vi "Device Settings.vi"(8 "error in":errorcluster, 11 "Class Objects In":T1) -> (0 "error out":errorcluster, 3 "Class Objects Out":T1)   [LabVIEW 2011]
uses:
  Controls/Class Objects.ctl
  Modules/File/Configuration/Configuration.lvclass
  Modules/Hardware/Mass Flow Controller/Mass Flow Controller.lvclass
  Modules/Hardware/Valve Controller/Valve Controller.lvclass
  Modules/Hardware/Power Supply/Power Supply.lvclass
  Modules/Hardware/Vapour Generator/Vapour Generator.lvclass
  Modules/Hardware/PID/PID.lvclass
  Modules/Hardware/Multimeter/Multimeter.lvclass
  Modules/File/TDMS/TDMS.lvclass
  Modules/Hardware/Power Supply/Source Mode.ctl
  Modules/Hardware/Power Supply/Source Units.ctl
  Modules/Hardware/Power Supply/Protection Limits.ctl
  Modules/Hardware/Power Supply/Voltage Units.ctl
  Modules/Hardware/Power Supply/Current Units.ctl
  Modules/Hardware/Aalborg GFC17/Flow Rate.ctl
  Modules/Hardware/Mass Flow Controller/Valve Status.ctl
  Modules/Hardware/Valve Controller/Valve Assembly.ctl
  Modules/Hardware/Valve Controller/Status.ctl
  Modules/Hardware/Agilent 3458A/Measurement Configuration.ctl
  Modules/Hardware/Agilent 3458A/Measurement Integration.ctl
  Modules/Hardware/Baseline Mocon piD-Tech plus/Settings.ctl
  Modules/Hardware/INL PID/Settings.ctl
  Modules/Hardware/Owlstone GEN-SYS/Permeation Tube.ctl
  Modules/Hardware/Owlstone GEN-SYS/Permeation Tube Gas.ctl
  Modules/Hardware/Owlstone GEN-SYS/Gen-Sys Setpoints.ctl
  Modules/Hardware/Vapour Generator/Gas Output.ctl
  Functional Global Data/Device Params Global.ctl
  Controls/Detector Type.ctl
  Controls/User Interface Action.ctl
  Controls/Devices.ctl
  Functional Global Data/Status Bar.ctl
  Modules/Hardware/Owlstone GEN-SYS/Owlstone GEN-SYS.lvclass
  Modules/Hardware/Agilent 3458A/Agilent 3458A.lvclass
  Modules/Hardware/Mass Flow Controller/Flow Rate Units.ctl
  Modules/Hardware/Valve Controller/Valves.ctl
  Modules/Hardware/Aalborg GFC17/Aalborg GFC17.lvclass
  Modules/Hardware/Baseline Mocon piD-Tech plus/Baseline Mocon piD-Tech plus.lvclass
  Modules/Hardware/INL PID/INL PID.lvclass
panel:
  in  "?":T2(tab)
  out "Gas Output":T3={"Concentration (ppm)"=inf, "Flow Rate (ml/min)"=0.0, "Relative Humidity (%)"=-1.0} {"Relative Humidity (%)" format="%#.4g"; "Flow Rate (ml/min)" format="%#.0f"; "Concentration (ppm)" format="%#.2g"}
  in  "Owlstone GEN-SYS Setpoints":T4={"OVG-4"={"Oven Temperature"=50, "Sample Flow Rate"=250, "Split Flow Status"=0, "Split Flow Rate"=0}, "OHG-4"={"Wet Air Flow"=500}} {"OHG-4"."Wet Air Flow" min=300 max=3000 scale=300.0..3000.0; "OVG-4"."Split Flow Status" items=["Closed", "Open"]; "OVG-4"."Split Flow Rate" min=300 max=3000 scale=50.0..3000.0; "OVG-4"."Sample Flow Rate" min=50 max=500 scale=50.0..500.0; "OVG-4"."Oven Temperature" min=25 max=100 scale=25.0..100.0}
  in  "Owlstone Permeation Tube":T5={"Tube"=enum."Ammonia 29 Sep 2012", "Molecular Weight"=56.106, "Calibration Temperature\n(Celcius)"=50, "Permeation Rate \n(ng/min)"=1539} {"Molecular Weight" min=0.0 format="%#.3g"; "Permeation Rate \n(ng/min)" min=0; "Calibration Temperature\n(Celcius)" min=0}
  in  "INL PID Settings":T7 caption="INL PID"
  in  "B-M PID Settings":T8 caption="Baseline Mocon piD-TECH plus"
  in  "Power Supply Output":bool caption="Output"
  in  "Power Supply Apply":bool
  in  "Power Supply Limits":T9 caption="Limits"
  in  "Power Supply Source Value Units":T12 caption="Source Value Units"
  in  "Power Supply Source Value":dbl caption="Source Value"
  in  "Power Supply Source Mode":T13 caption="Source Mode"
  in  "Agilent 3458A Measurement Integration":T14={"Power Line Cycles"=10.0} caption="Measurement Integration"
  in  "Agilent 3458A Multimeter Measurement Configuration":T15 caption="Measurement Configuration"
  in  "MFC Valve Status":T16=enum."Closed" caption="Valve Status"
  in  "MFC Flow Rate":T17 caption="Flow Rate" min=0.0 max=200.0 scale=0.0..200.0
  in  "Valves Open All":bool
  in  "Valves Close All":bool
  in  "Valve Assembly":T18 {"Valve 5" items=["Closed", "Open"]; "Valve 4" items=["Closed", "Open"]; "Valve 3" items=["Closed", "Open"]; "Valve 2" items=["Closed", "Open"]; "Valve 1" items=["Closed", "Open"]}
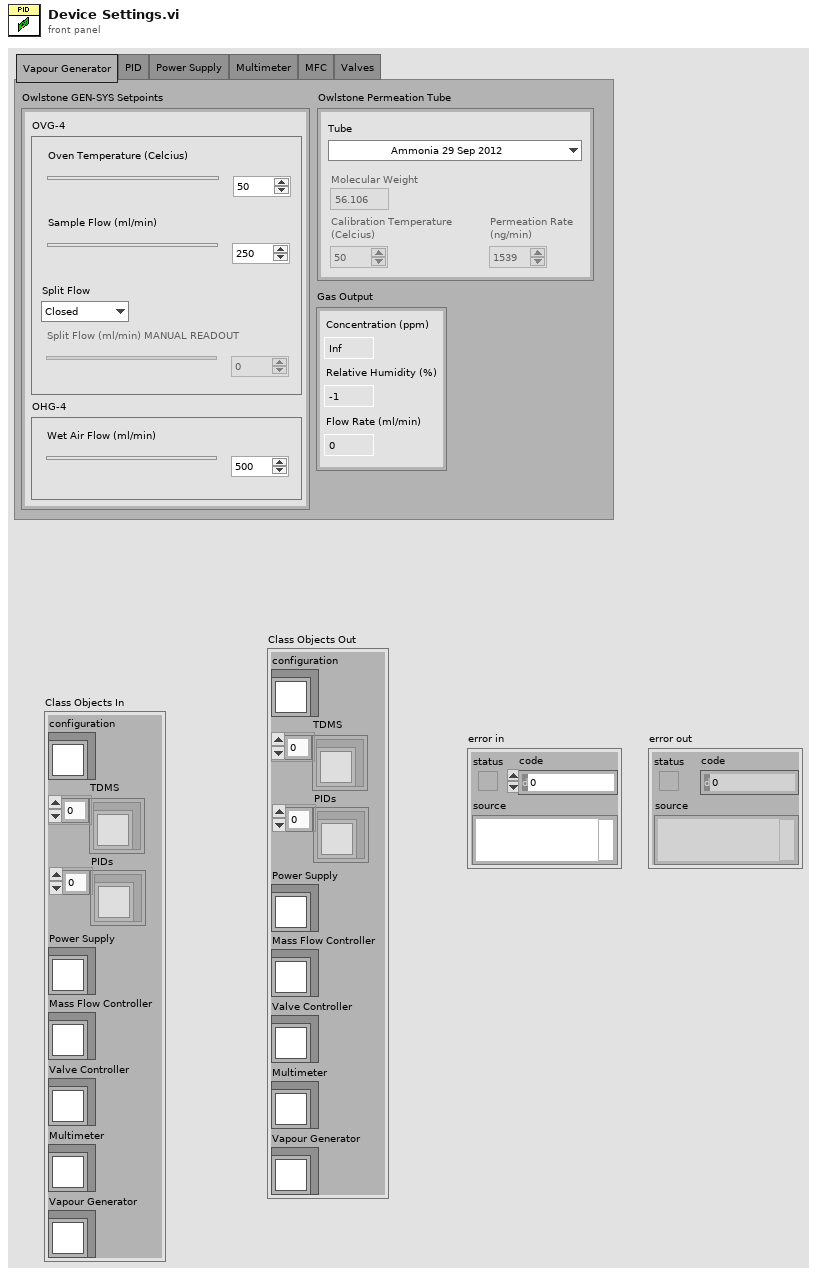
[diagram p1: front panel]
types:
  T1 = typedef "Class Objects.ctl" = cluster{"configuration":refnum<class "Configuration.lvclass">, "TDMS":refnum<class "TDMS.lvclass">[], "Power Supply":refnum<class "Power Supply.lvclass">, "Mass Flow Controller":refnum<class "Mass Flow Controller.lvclass">, "Valve Controller":refnum<class "Valve Controller.lvclass">, "Multimeter":refnum<class "Multimeter.lvclass">, "Vapour Generator":refnum<class "Vapour Generator.lvclass">, "PIDs":refnum<class "PID.lvclass">[]}
  T2 = enum32{"Vapour Generator", "PID", "Power Supply", "Multimeter", "MFC", "Valves"}
  T3 = typedef "Vapour Generator.lvclass/Gas Output.ctl" = cluster{"Concentration (ppm)":dbl, "Flow Rate (ml/min)":dbl, "Relative Humidity (%)":dbl}
  T4 = typedef "Owlstone GEN-SYS.lvclass/Gen-Sys Setpoints.ctl" = cluster{"OVG-4":cluster{"Oven Temperature":i32, "Sample Flow Rate":i32, "Split Flow Status":u16, "Split Flow Rate":i32}, "OHG-4":cluster{"Wet Air Flow":i32}}
  T5 = typedef "Owlstone GEN-SYS.lvclass/Permeation Tube.ctl" = cluster{"Tube":T6, "Molecular Weight":dbl, "Calibration Temperature\n(Celcius)":i32, "Permeation Rate \n(ng/min)":i32}
  T6 = typedef "Owlstone GEN-SYS.lvclass/Permeation Tube Gas.ctl" = enum16{"Isobutylene 27 Nov 2012", "Ammonia 29 Sep 2012", "DMMP Tube A 3 July 2014", "DMMP Tube B 3 July 2014"}
  T7 = typedef "INL PID.lvclass/Settings.ctl" = cluster{"Sampling Frequency":dbl, "Integration Time":dbl, "Integration Periods":u8, "Grid Voltage":dbl}
  T8 = typedef "Baseline Mocon piD-Tech plus.lvclass/Settings.ctl" = cluster{"Detector Sampling Frequency":dbl}
  T9 = typedef "Power Supply.lvclass/Protection Limits.ctl" = cluster{"Voltage Limit":dbl, "Voltage Limit Units":T10, "Current Limit":dbl, "Current Limit Units":T11, "Voltage Trip/Cmpl":dbl, "Voltage Trip/Cmpl Units":T10, "Current Trip/Cmpl":dbl, "Current Trip/Cmpl Units":T11}
  T10 = typedef "Power Supply.lvclass/Voltage Units.ctl" = enum16{"volts", "millivolts", "microvolts"}
  T11 = typedef "Power Supply.lvclass/Current Units.ctl" = enum16{"amps", "milliamps", "microamps", "nanoamps"}
  T12 = typedef "Power Supply.lvclass/Source Units.ctl" = enum16{"volts", "millivolts", "microvolts", "amps", "milliamps", "microamps", "nanoamps"}
  T13 = typedef "Power Supply.lvclass/Source Mode.ctl" = enum16{"Volts", "Current"}
  T14 = typedef "Agilent 3458A.lvclass/Measurement Integration.ctl" = cluster{"Power Line Cycles":dbl}
  T15 = typedef "Agilent 3458A.lvclass/Measurement Configuration.ctl" = cluster{"Function":enum16{"DC Voltage", "AC Voltage", "AC + DC Voltage", "DC Current", "AC Current", "AC + DC Current", "2-Wire Resistance", "4-Wire Resistance", "Frequency", "Period", "Direct Sampling DC", "Direct Sampling AC", "Sub-Sampling DC", "Sub-Sampling AC"}, " Manual Resolution":enum16{"4.5", "5.5", "6.5", "7.5", "8.5"}, "Frequency Source":enum16{"AC + DC Current", "AC + DC Voltage", "AC Current", "AC Voltage"}, "Auto Range":enum16{"OFF", "ON", "ONCE"}}
  T16 = typedef "Mass Flow Controller.lvclass/Valve Status.ctl" = enum16{"Open", "Closed"}
  T17 = typedef "Aalborg GFC17.lvclass/Flow Rate.ctl" = dbl
  T18 = typedef "Valve Controller.lvclass/Valve Assembly.ctl" = cluster{"Valve 1":T19, "Valve 2":T19, "Valve 3":T19, "Valve 4":T19, "Valve 5":T19}
  T19 = typedef "Valve Controller.lvclass/Status.ctl" = u16
  T20 = typedef "Device Params Global.ctl" = enum16{"Initialize", "Get Device Settings", "Get Device Connections", "Set Device Settings", "Set Device Connections", "Get All Device Properties"}
  T21 = typedef "Device Connections.ctl" = cluster{"Detector":cluster{"Detector Type":T22, "Connection":bool, "B-M PID":T23, "INL PID Connections":T24}, "Power Supply":cluster{"Type":enum16{"Stanford Research PS350", "Keithley 2400"}, "Connection":bool, "VISA resource name":refnum<visa-resource-name>}, "Mass Flow Controller":cluster{"Type":enum16{"Aalborg GFC17"}, "Connection":bool, "Aalborg GFC17":T26}, "Valve Controller":cluster{"Type":T27, "Connection":bool, "SMC - INL":cluster{"VISA resource name":refnum<visa-resource-name>}}, "Multimeter":cluster{"Multimeter Type":T28, "Connection":bool, "VISA resource name":refnum<visa-resource-name>}, "Vapour Generator":cluster{"Type":T29, "Connection":bool, "Owlstone Gen-SYS":T30}}
  T22 = typedef "Detector Type.ctl" = enum16{"INL PID", "Baseline-Mocon piD-TECH plus"}
  T23 = typedef "Baseline Mocon piD-Tech plus.lvclass/Connections.ctl" = cluster{"AI DAQmx channel":tag}
  T24 = typedef "INL PID Connections.ctl" = cluster{"PIDs":u8, "Integrator DAQ Channels 1":T25, "Integrator DAQ Channels 2":T25}
  T25 = typedef "INL PID.lvclass/Integrator DAQmx Channels.ctl" = cluster{"V0":tag, "S1":tag, "S2":tag}
  T26 = typedef "Aalborg GFC17.lvclass/Aalborg GFC17 Connections.ctl" = cluster{"flow rate setpoint channel":tag, "flow rate reading channel":tag, "valve channel":tag}
  T27 = typedef "Valve Type.ctl" = enum16{"SMC - INL"}
  T28 = typedef "Multimeter Type.ctl" = enum16{"Agilent 3458A"}
  T29 = typedef "Vapour Generator Type.ctl" = enum16{"Owlstone GEN-SYS"}
  T30 = typedef "Owlstone GEN-SYS.lvclass/GEN-SYS Connections.ctl" = cluster{"GEN-SYS VISA resource name":refnum<visa-resource-name>, "OVG-4":cluster{"Flow Address":u8, "Temp Address":u8}, "OHG-4":cluster{"Flow Address":u8, "Easydew VISA resource name":refnum<visa-resource-name>}}
  T31 = typedef "Device Settings.ctl" = cluster{"PID":cluster{"B-M PID":T8, "INL PID":T7}, "Power Supply":cluster{"Source Value":dbl, "Source Value Units":T12, "Source Mode":T13, "Limits":T9, "Output":bool}, "Mass Flow Controller":cluster{"MFC Flow Rate":dbl, "MFC Valve Status":T16}, "Valve Controller":cluster{"Valve Assembly":T18}, "Multimeter":cluster{"Agilent 3458A":cluster{"Measurement Configuration":T15, "Measurement Integration":T14}}, "Vapour Generator":cluster{"Owlstone Permeation Tube":T5, "Owlstone GEN-SYS Setpoints":T4}}
  T32 = enum8{"Enabled", "Disabled", "Disabled and Grayed Out"}
  T33 = cluster{"Valve 1":T19, "Valve 2":T19, "Valve 3":T19, "Valve 4":T19, "Valve 5":T19}
  T34 = typedef "User Interface Action.ctl" = enum16{"Initialize", "Data Acquisition Disable", "Data View Disable", "Sample Set", "Sample Set 2D Data", "Sample Set x0 & dx", "Sample Add", "Sample Set Cursor", "Sample Set Offset & Multiplier", "Sample Set Axis Labels", "Sample Parameters Disabled", "Sample Parameters Update", "Run Update", "Run Set Offset & Multiplier", "Run Set Axis Labels", "Run Set Cursor", "Run Set Disabled", "Run Parameters Update", "Run Parameters Disabled", "Run Number Set", "Run Number Set Range", "Run Number Set Disabled", "Sample Number Set", "Sample Number Set Range", "Notes Set Value", "Update Plot", "Set Plot Parameters", "Update Concentration Plot", "Time Set", "Clear DAQ Display", "Clear Analysis Display", "Status Bar Set", "Progress Bar Set", "Display Mode Set", "Experiment Type Set", "Analysis Plot Average Set", "Stop"}
  T35 = typedef "Devices.ctl" = enum16{"Detector", "Mass Flow Controller", "Power Supply"}
  T36 = typedef "Status Bar.ctl" = enum16{"Insert Into Status Bar", "Get Status Bar", "Initialize"}
  T37 = typedef "Mass Flow Controller.lvclass/Flow Rate Units.ctl" = enum16{"ml/min"}
  T38 = enum16{"Stanford Research PS350", "Keithley 2400"}
  T39 = cluster{"Tube":T6, "Molecular Weight":dbl, "Calibration Temperature\n(Celcius)":i32, "Permeation Rate \n(ng/min)":i32}
  T40 = typedef "Valve Controller.lvclass/Valves.ctl" = u16
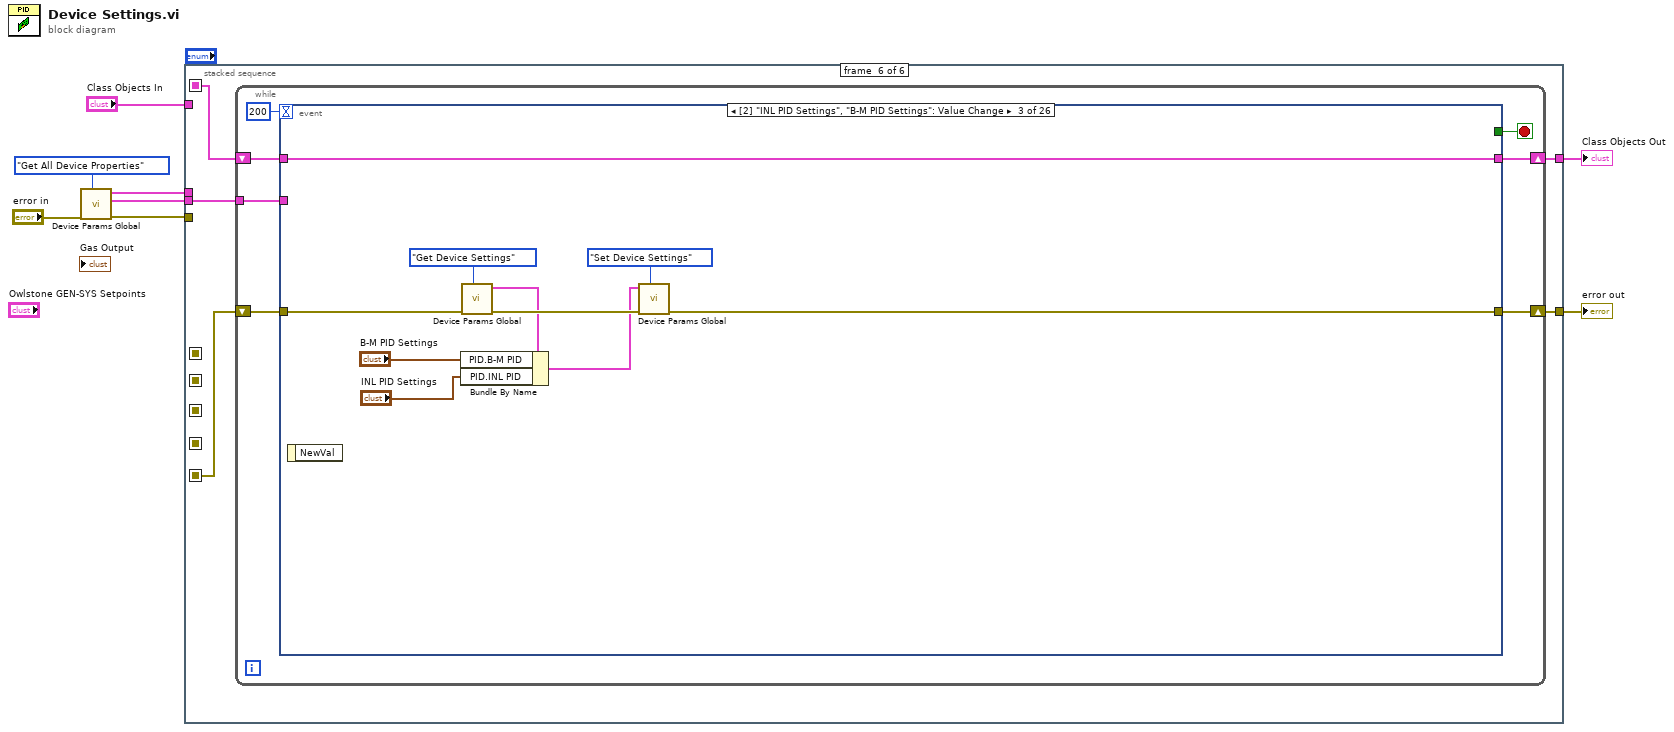
[diagram p0: block diagram]
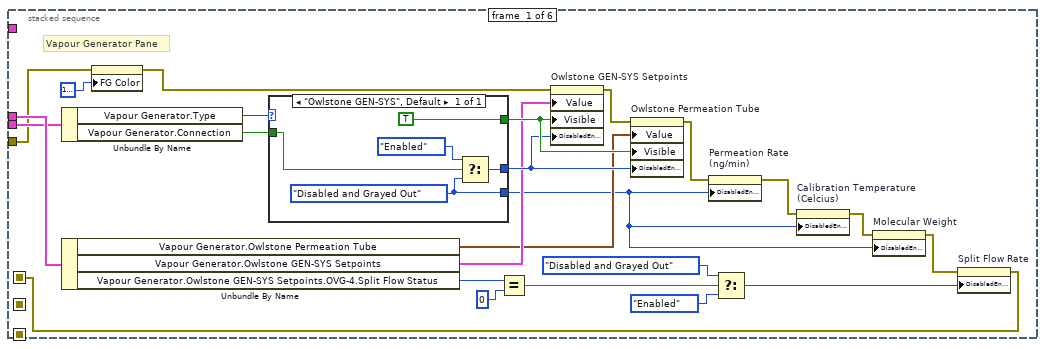
[diagram p2: hidden frame]
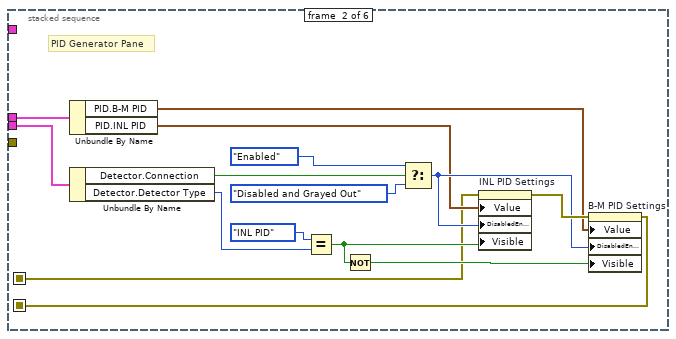
[diagram p3: hidden frame]
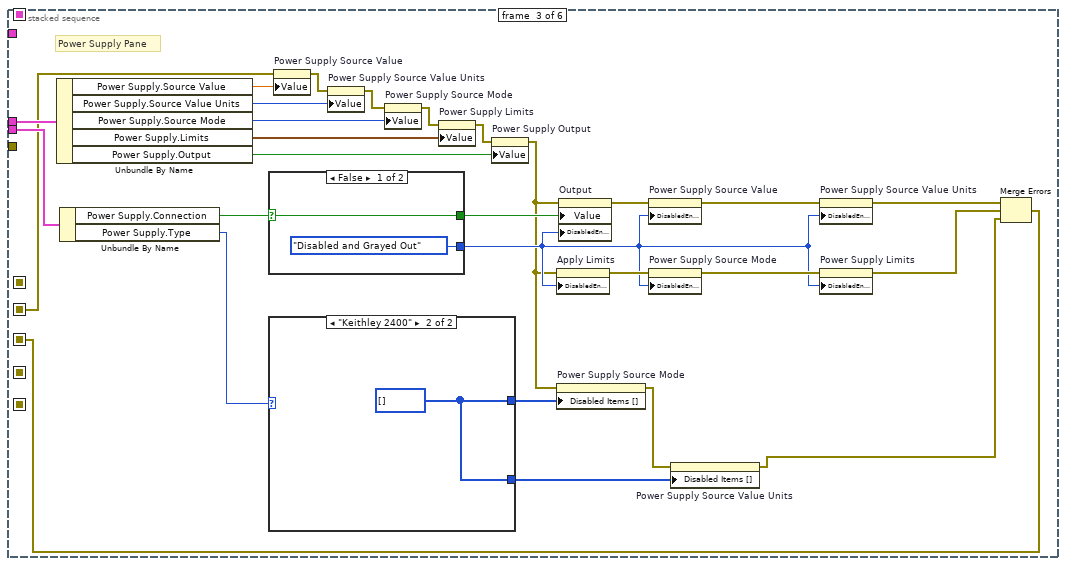
[diagram p4: hidden frame]
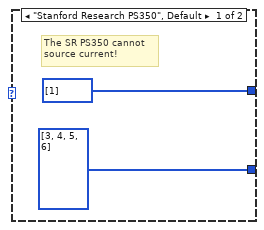
[diagram p5: hidden frame]
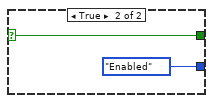
[diagram p6: hidden frame]
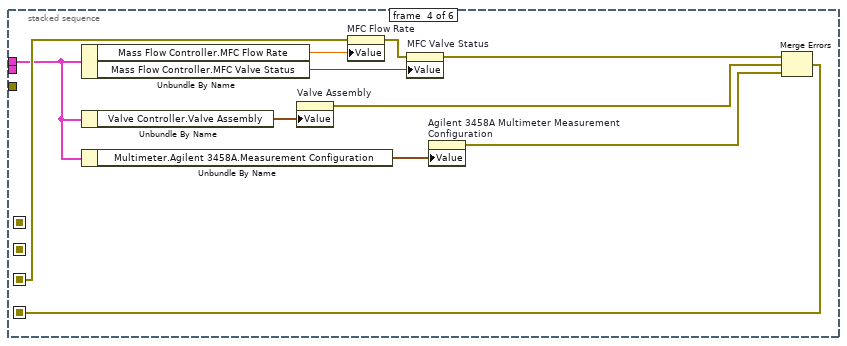
[diagram p7: hidden frame]
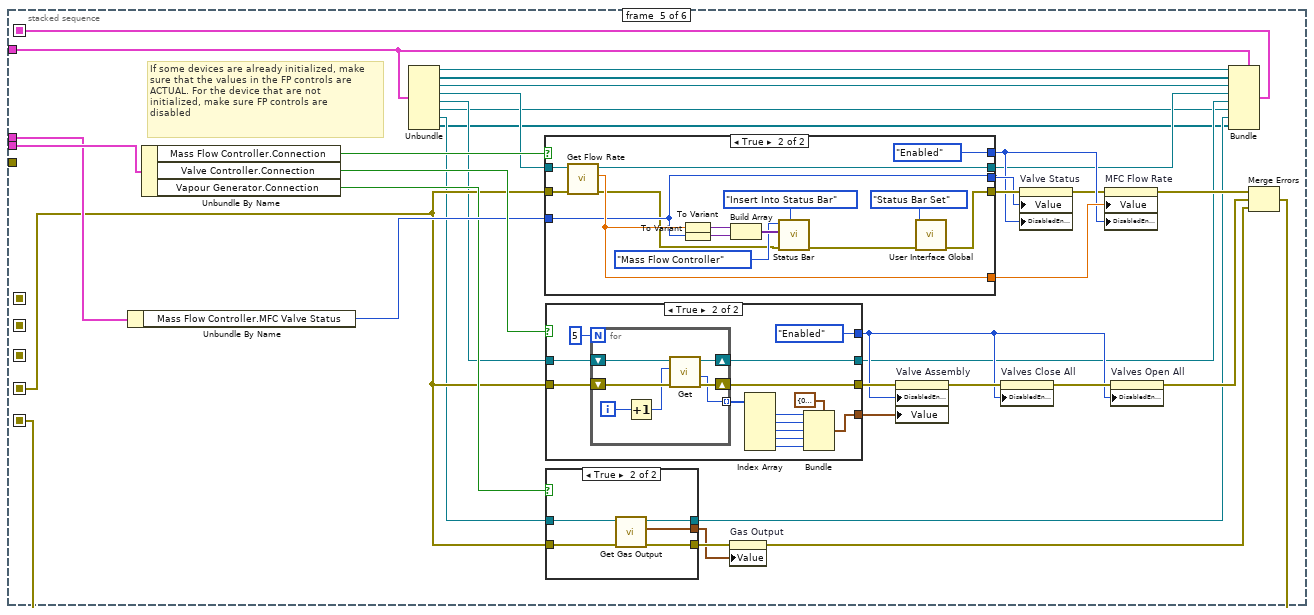
[diagram p8: hidden frame]
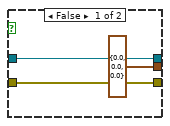
[diagram p9: hidden frame]
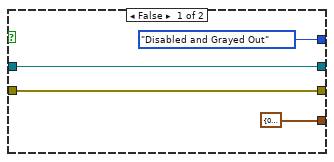
[diagram p10: hidden frame]
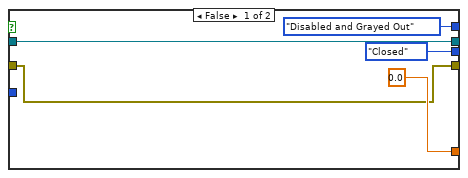
[diagram p11: hidden frame]
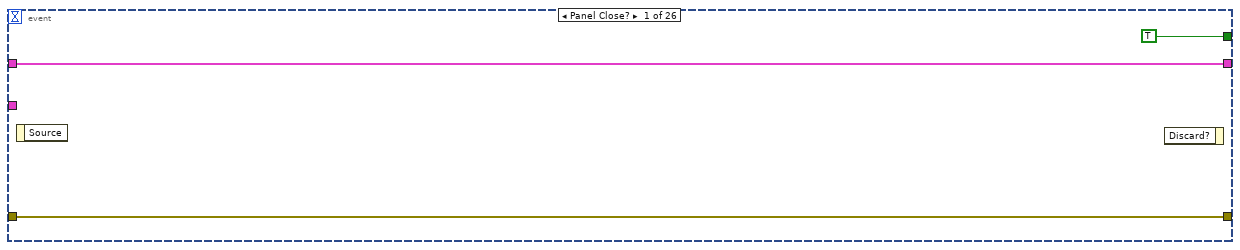
[diagram p12: hidden frame]
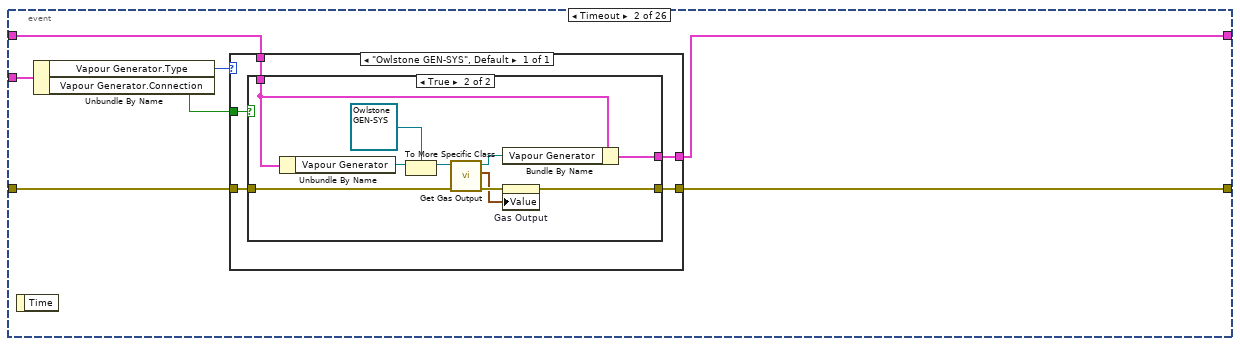
[diagram p13: hidden frame]
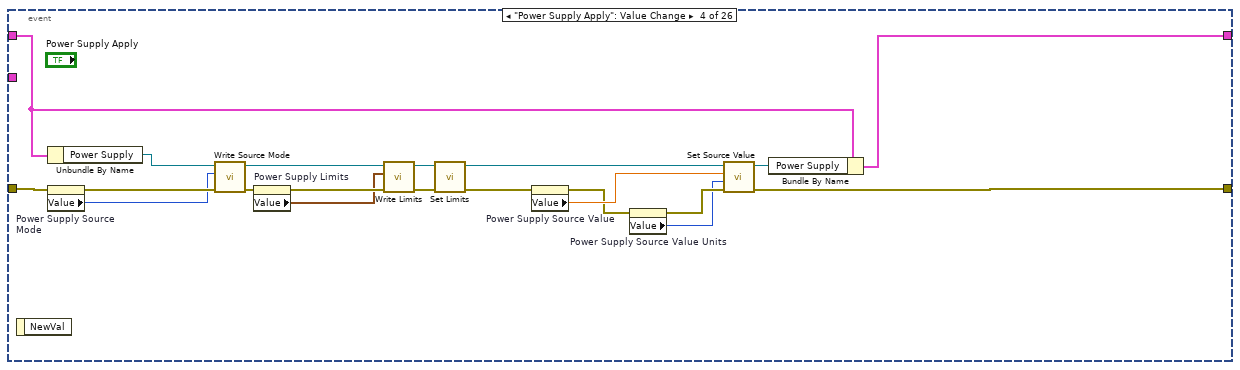
[diagram p15: hidden frame]
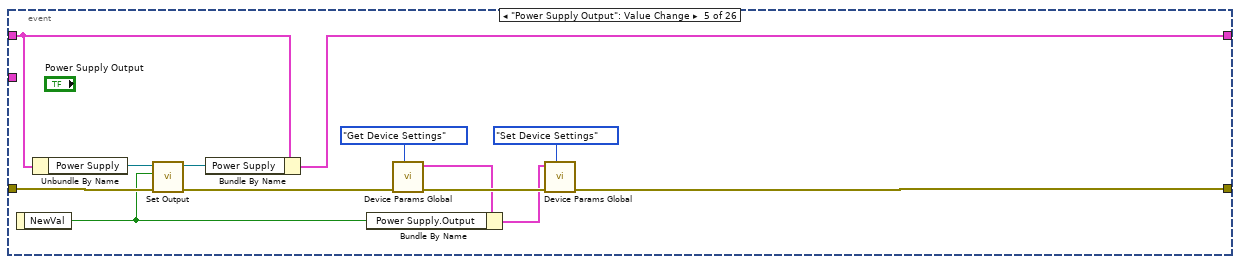
[diagram p16: hidden frame]
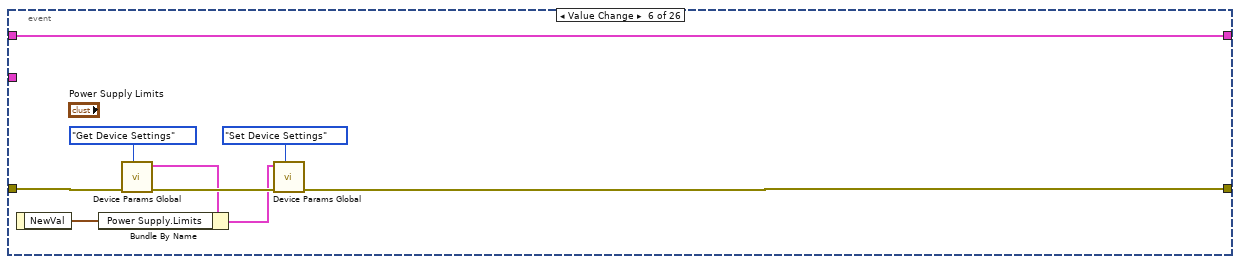
[diagram p17: hidden frame]
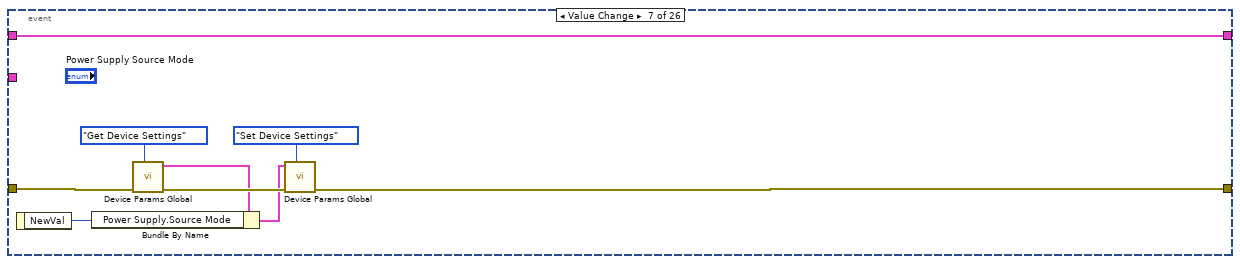
[diagram p18: hidden frame]
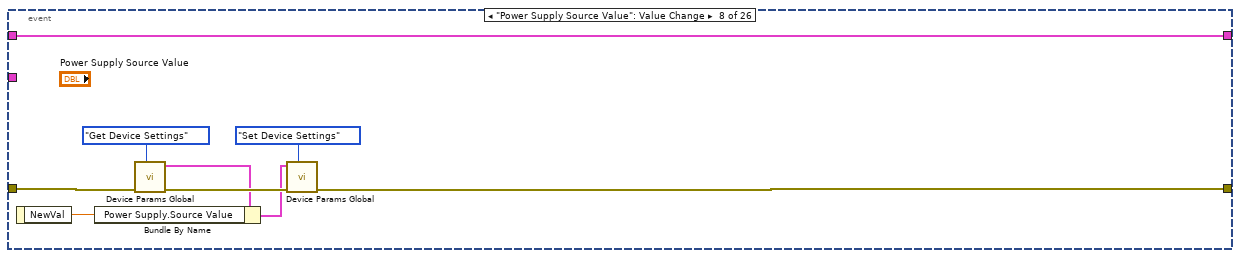
[diagram p19: hidden frame]
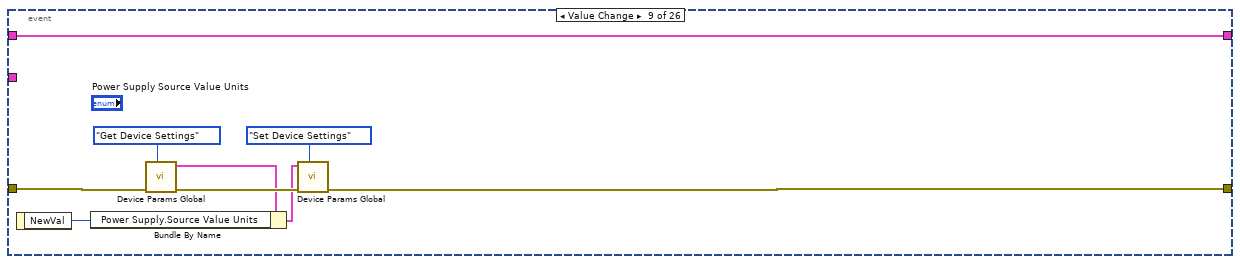
[diagram p20: hidden frame]
diagram:
  n1 = call "Device Params Global.vi"("action"=Device_Params_Global."Get All Device Properties", "error in"="error in") -> ("error out"=w4:errorcluster, "Device Connections OUT"=w2:T21, "Device Settings OUT"=w1:T31)  [unwired: 7 in]
  n2 = stacked-sequence {
    seq-local: [w9 _ _ _ _ _] -> [_ w39 _ _ _ _]
    seq-local: [_ _ _ _ w132 _] -> [_ _ _ _ _ w190]
    seq-local: [_ _ w53 _ _ _] -> [_ _ _ w90 _ _]
    seq-local: [_ w38 _ _ _ _] -> [_ _ w60 _ _ _]
    seq-local: [_ _ _ w88 _ _] -> [_ _ _ _ w110 _]
    seq-local: [_ _ _ _ w111 _] -> [_ _ _ _ _ w189]
    tunnel: [_ _ _ _ _ w191] -> w8
    tunnel: w4 -> [w13 _ _ _ _ _]
    tunnel: "Class Objects In" -> [_ _ _ _ w134 _]
    tunnel: [_ _ _ _ _ w192] -> w6
    tunnel: w2 -> [w31 w42 w64 _ w113 w188]
    tunnel: w1 -> [w32 w43 w71 w89 w112 _]
    frame #0 {
      # "Vapour Generator Pane"
      n3 = Unbundle By Name(w31) -> ("Vapour Generator.Type"=w30:T29, "Vapour Generator.Connection"=w29:bool)
      n4 = Unbundle By Name(w32) -> ("Vapour Generator.Owlstone Permeation Tube"=w25:T5, "Vapour Generator.Owlstone GEN-SYS Setpoints"=w26:T4, "Vapour Generator.Owlstone GEN-SYS Setpoints.OVG-4.Split Flow Status"=w18:u16)
      n5 = property class="TabCtl (strict)"(error in=w13, "FG Color"=u32 16777238) -> (error out=w12:errorcluster)  [unwired: 1 in, 1 out]
      n6 = case shown="\"Owlstone GEN-SYS\", Default" w30 {
        tunnel: [TRUE] -> w28
        tunnel: w29 -> [w35]
        tunnel: [w34] -> w27
        tunnel: [w33] -> w19
        frame "Owlstone GEN-SYS", Default {
          w33 = T32."Disabled and Grayed Out" ("Disabled")
          n7 = Select(t=T32."Enabled" ("Disabled"), s=w35, f=w33) -> (s? t:f=w34:T32)
        }
      }
      n8 = Equal?(x=w18, y=u16 0) -> (x = y?=w16:bool)
      n9 = property on="Owlstone GEN-SYS Setpoints" class="Clust (strict)"(error in=w12, "Value"=w26, "Visible"=w28, "DisabledEnum"=w27) -> (error out=w24:errorcluster)  [unwired: 1 in, 1 out]
      n10 = property on="Owlstone Permeation Tube" class="Clust (strict)"(error in=w24, "Value"=w25, "Visible"=w28, "DisabledEnum"=w27) -> (error out=w20:errorcluster)  [unwired: 1 in, 1 out]
      n11 = property on="Permeation Rate \n(ng/min)" class="DigNum (strict)"(error in=w20, "DisabledEnum"=w19) -> (error out=w22:errorcluster)  [unwired: 1 in, 1 out]
      n12 = Select(t=T32."Disabled and Grayed Out" ("Disabled"), s=w16, f=T32."Enabled" ("Disabled")) -> (s? t:f=w11:T32)
      n13 = property on="Calibration Temperature\n(Celcius)" class="DigNum (strict)"(error in=w22, "DisabledEnum"=w19) -> (error out=w21:errorcluster)  [unwired: 1 in, 1 out]
      n14 = property on="Molecular Weight" class="DigNum (strict)"(error in=w21, "DisabledEnum"=w19) -> (error out=w10:errorcluster)  [unwired: 1 in, 1 out]
      n15 = property on="Split Flow Rate" class="Slide (strict)"(error in=w10, "DisabledEnum"=w11) -> (error out=w9:errorcluster)  [unwired: 1 in, 1 out]
    }
    frame #1 {
      # "PID Generator Pane"
      n16 = Unbundle By Name(w43) -> ("PID.B-M PID"=w40:T8, "PID.INL PID"=w41:T7)
      n17 = Unbundle By Name(w42) -> ("Detector.Connection"=w52:bool, "Detector.Detector Type"=w47:T22)
      n18 = Equal?(x=Detector_Type."INL PID" ("y"), y=w47) -> (x = y?=w45:bool)
      n19 = Not(x=w45) -> (.not. x?=w44:bool)
      n20 = Select(t=T32."Enabled" ("Disabled"), s=w52, f=T32."Disabled and Grayed Out" ("Disabled")) -> (s? t:f=w48:T32)
      n21 = property on="INL PID Settings" class="Clust (strict)"(error in=w39, "Value"=w41, "DisabledEnum"=w48, "Visible"=w45) -> (error out=w49:errorcluster)  [unwired: 1 in, 1 out]
      n22 = property on="B-M PID Settings" class="Clust (strict)"(error in=w49, "Value"=w40, "DisabledEnum"=w48, "Visible"=w44) -> (error out=w38:errorcluster)  [unwired: 1 in, 1 out]
    }
    frame #2 {
      # "Power Supply Pane"
      n23 = Unbundle By Name(w71) -> ("Power Supply.Source Value"=w80:dbl, "Power Supply.Source Value Units"=w79:T12, "Power Supply.Source Mode"=w77:T13, "Power Supply.Limits"=w74:T9, "Power Supply.Output"=w72:bool)
      n24 = Unbundle By Name(w64) -> ("Power Supply.Connection"=w63:bool, "Power Supply.Type"=w57:T38)
      n25 = case shown="False" w63 {
        selector: w63 -> [w84 w86]
        tunnel: [T32."Disabled and Grayed Out" ("Disabled") T32."Enabled" ("Disabled")] -> w65
        tunnel: [w84 w86] -> w70
        frame False {
        }
        frame True {
        }
      }
      n26 = case shown="\"Keithley 2400\"" w57 {
        tunnel: [i32[] [1] ("Disabled Items []") w83] -> w59
        tunnel: [i32[] [3, 4, 5, 6] ("Disabled Items []") w83] -> w58
        frame "Stanford Research PS350", Default {
          # "The SR PS350 cannot \nsource current!"
        }
        frame "Keithley 2400" {
          w83 = i32[] [] ("Disabled Items []")
        }
      }
      n27 = property on="Power Supply Source Value" class="DigNum (strict)"(error in=w60, "Value"=w80) -> (error out=w78:errorcluster)  [unwired: 1 in, 1 out]
      n28 = property on="Power Supply Source Value Units" class="Enum (strict)"(error in=w78, "Value"=w79) -> (error out=w76:errorcluster)  [unwired: 1 in, 1 out]
      n29 = property on="Power Supply Source Mode" class="Enum (strict)"(error in=w76, "Value"=w77) -> (error out=w75:errorcluster)  [unwired: 1 in, 1 out]
      n30 = property on="Power Supply Limits" class="Clust (strict)"(error in=w75, "Value"=w74) -> (error out=w73:errorcluster)  [unwired: 1 in, 1 out]
      n31 = property on="Power Supply Output" class="Bool (strict)"(error in=w73, "Value"=w72) -> (error out=w56:errorcluster)  [unwired: 1 in, 1 out]
      n32 = property on="Apply Limits" class="Bool"(error in=w56, "DisabledEnum"=w65) -> (error out=w67:errorcluster)  [unwired: 1 in, 1 out]
      n33 = property on="Power Supply Source Mode" class="Enum (strict)"(error in=w56, "Disabled Items []"=w59) -> (error out=w55:errorcluster)  [unwired: 1 in, 1 out]
      n34 = property on="Output" class="Bool (strict)"(error in=w56, "Value"=w70, "DisabledEnum"=w65) -> (error out=w69:errorcluster)  [unwired: 1 in, 1 out]
      n35 = property on="Power Supply Source Value" class="DigNum (strict)"(error in=w69, "DisabledEnum"=w65) -> (error out=w68:errorcluster)  [unwired: 1 in, 1 out]
      n36 = property on="Power Supply Source Mode" class="Enum (strict)"(error in=w67, "DisabledEnum"=w65) -> (error out=w66:errorcluster)  [unwired: 1 in, 1 out]
      n37 = property on="Power Supply Source Value Units" class="Enum (strict)"(error in=w55, "Disabled Items []"=w58) -> (error out=w54:errorcluster)  [unwired: 1 in, 1 out]
      n38 = property on="Power Supply Source Value Units" class="Enum (strict)"(error in=w68, "DisabledEnum"=w65) -> (error out=w62:errorcluster)  [unwired: 1 in, 1 out]
      n39 = property on="Power Supply Limits" class="Clust (strict)"(error in=w66, "DisabledEnum"=w65) -> (error out=w61:errorcluster)  [unwired: 1 in, 1 out]
      n40 = Merge Errors(w62, w61, w54) -> (w53:errorcluster)
    }
    frame #3 {
      n41 = Unbundle By Name(w89) -> ("Mass Flow Controller.MFC Flow Rate"=w97:dbl, "Mass Flow Controller.MFC Valve Status"=w96:T16)
      n42 = Unbundle By Name(w89) -> ("Valve Controller.Valve Assembly"=w95:T18)
      n43 = Unbundle By Name(w89) -> ("Multimeter.Agilent 3458A.Measurement Configuration"=w92:T15)
      n44 = property on="Valve Assembly" class="Clust (strict)"("Value"=w95) -> (error out=w93:errorcluster)  [unwired: 2 in, 1 out]
      n45 = property on="MFC Flow Rate" class="Slide (strict)"(error in=w90, "Value"=w97) -> (error out=w98:errorcluster)  [unwired: 1 in, 1 out]
      n46 = property on="MFC Valve Status" class="Enum (strict)"(error in=w98, "Value"=w96) -> (error out=w94:errorcluster)  [unwired: 1 in, 1 out]
      n47 = property on="Agilent 3458A Multimeter Measurement Configuration" class="Clust (strict)"("Value"=w92) -> (error out=w91:errorcluster)  [unwired: 2 in, 1 out]
      n48 = Merge Errors(w94, w93, w91) -> (w88:errorcluster)
    }
    frame #4 {
      # "If some devices are already initialized, make \nsure that the values in the FP controls are \nACTUAL. For the device that are not \ninitialized, make sure FP controls are \ndisabled"
      n49 = Unbundle By Name(w112) -> ("Mass Flow Controller.MFC Valve Status"=w116:T16)
      n50 = Unbundle By Name(w113) -> ("Mass Flow Controller.Connection"=w130:bool, "Valve Controller.Connection"=w119:bool, "Vapour Generator.Connection"=w115:bool)
      n51 = Unbundle(w134) -> ("configuration"=w114:refnum<class "Configuration.lvclass">, "TDMS"=w133:refnum<class "TDMS.lvclass">[], "Power Supply"=w131:refnum<class "Power Supply.lvclass">, "Mass Flow Controller"=w106:refnum<class "Mass Flow Controller.lvclass">, "Valve Controller"=w104:refnum<class "Valve Controller.lvclass">, "Multimeter"=w99:refnum<class "Multimeter.lvclass">, "Vapour Generator"=w102:refnum<class "Vapour Generator.lvclass">, "PIDs"=w100:refnum<class "PID.lvclass">[])
      n52 = case shown="True" w130 {
        tunnel: [w168 w180] -> w129
        tunnel: w106 -> [w172 w179]
        tunnel: [Valve_Status."Closed" ("Valve Status") w176] -> w128
        tunnel: [0.0 ("Flow Rate") w178] -> w127
        tunnel: [w172 w175] -> w105
        tunnel: [T32."Disabled and Grayed Out" ("Disabled") T32."Enabled" ("Disabled")] -> w126
        tunnel: w116 -> [_ w176]
        tunnel: w110 -> [w168 w173]
        frame False {
        }
        frame True {
          n53 = call-dynamic "Get Flow Rate.vi"("error in (no error)"=w173, "Mass Flow Controller in"=w179) -> ("error out"=w174:errorcluster, "Flow Rate"=w178:dbl, "Mass Flow Controller out"=w175:refnum<class "Mass Flow Controller.lvclass">)  [unwired: 6 in, 1 out]
          n54 = To Variant(anything=w178) -> (Variant=w187:variant)
          n55 = To Variant(anything=w176) -> (Variant=w186:variant)
          n56 = Build Array(w187, w186) -> (w185:variant[])
          n57 = call "Status Bar.vi"("action"=Status_Bar."Insert Into Status Bar", "error in"=w174, "Parameters"=w185, "Devices"=Devices."Mass Flow Controller") -> ("error out"=w181:errorcluster)  [unwired: 6 in, 1 out]
          n58 = call "User Interface Global.vi"("error in"=w181, "action"=User_Interface_Action."Status Bar Set") -> ("error out"=w180:errorcluster)  [unwired: 9 in]
        }
      }
      n59 = case shown="True" w119 {
        tunnel: w104 -> [w146 w160]
        tunnel: [w146 w150] -> w103
        tunnel: [w143 w151] -> w122
        tunnel: [T33 {"Valve 1"=0, "Valve 2"=0, "Valve 3"=0, "Valve 4"=0, "Valve 5"=0} ("Valve Assembly") w149] -> w121
        tunnel: [T32."Disabled and Grayed Out" ("Disabled") T32."Enabled" ("Disabled")] -> w117
        tunnel: w110 -> [w143 w147]
        frame False {
        }
        frame True {
          n60 = for {
            N: 5 -> [_]
            shift-right: [w164] -> w150
            shift-left: w160 -> [w165]
            shift-right: [w166] -> w151
            shift-left: w147 -> [w167]
            tunnel: [w161] -> w157 mode=indexing
            i -> [w163]
            n61 = Increment(x=w163) -> (x+1=w162:i32)
            n62 = call-dynamic "Get.vi"("error in (no error)"=w167, "valve in"=w162, "Valve Controller in"=w165) -> ("error out"=w166:errorcluster, "status out"=w161:T19, "Valve Controller out"=w164:refnum<class "Valve Controller.lvclass">)  [unwired: 5 in, 1 out]
          }
          n63 = Index Array(array=w157) -> (element #1=w156:T19, element #2=w155:T19, element #3=w154:T19, element #4=w153:T19, element #5=w152:T19)  [unwired: 5 in]
          n64 = Bundle(cluster=T33 {"Valve 1"=0, "Valve 2"=0, "Valve 3"=0, "Valve 4"=0, "Valve 5"=0} ("Valve Assembly"), "Valve 1"=w156, "Valve 2"=w155, "Valve 3"=w154, "Valve 4"=w153, "Valve 5"=w152) -> (w149:T33)
        }
      }
      n65 = case shown="True" w115 {
        tunnel: w102 -> [w137 w142]
        tunnel: [w137 w141] -> w101
        tunnel: w110 -> [w136 w140]
        tunnel: [w136 w139] -> w109
        tunnel: [T3 {"Concentration (ppm)"=0.0, "Flow Rate (ml/min)"=0.0, "Relative Humidity (%)"=0.0} ("Output") w138] -> w107
        frame False {
        }
        frame True {
          n66 = call-dynamic "Get Gas Output.vi"("error in (no error)"=w140, "Vapour Generator in"=w142) -> ("error out"=w139:errorcluster, "Output"=w138:T3, "Vapour Generator out"=w141:refnum<class "Vapour Generator.lvclass">)  [unwired: 7 in]
        }
      }
      n67 = property on="Gas Output" class="Clust (strict)"(error in=w109, "Value"=w107) -> (error out=w108:errorcluster)  [unwired: 1 in, 1 out]
      n68 = property on="Valve Assembly" class="Clust (strict)"(error in=w122, "DisabledEnum"=w117, "Value"=w121) -> (error out=w123:errorcluster)  [unwired: 1 in, 1 out]
      n69 = property on="Valves Close All" class="Bool"(error in=w123, "DisabledEnum"=w117) -> (error out=w120:errorcluster)  [unwired: 1 in, 1 out]
      n70 = property on="Valve Status" class="Enum (strict)"(error in=w129, "Value"=w128, "DisabledEnum"=w126) -> (error out=w125:errorcluster)  [unwired: 1 in, 1 out]
      n71 = property on="MFC Flow Rate" class="Slide (strict)"(error in=w125, "Value"=w127, "DisabledEnum"=w126) -> (error out=w124:errorcluster)  [unwired: 1 in, 1 out]
      n72 = property on="Valves Open All" class="Bool"(error in=w120, "DisabledEnum"=w117) -> (error out=w118:errorcluster)  [unwired: 1 in, 1 out]
      n73 = Bundle(cluster=w134, "configuration"=w114, "TDMS"=w133, "Power Supply"=w131, "Mass Flow Controller"=w105, "Valve Controller"=w103, "Multimeter"=w99, "Vapour Generator"=w101, "PIDs"=w100) -> (w132:T1)
      n74 = Merge Errors(w124, w118, w108) -> (w111:errorcluster)
    }
    frame #5 {
      n75 = while {
        shift-right: [w195] -> w192
        shift-left: w190 -> [w198]
        shift-right: [w196] -> w191
        shift-left: w189 -> [w197]
        tunnel: w188 -> [w193]
        stop <- w199 stop-if-true
        n76 = event shown="[2] \"INL PID Settings\", \"B-M PID Settings\": Value Change" {
          selector: _ -> [_ _ _ _ _ _ _ _ _ _ _ _ _ _ _ _ _ _ _ _ _ _ _ _ _ _]
          dyn-events: _ -> [_ _ _ _ _ _ _ _ _ _ _ _ _ _ _ _ _ _ _ _ _ _ _ _ _ _]
          timeout: 200 -> [_ _ _ _ _ _ _ _ _ _ _ _ _ _ _ _ _ _ _ _ _ _ _ _ _ _]
          tunnel: [w201 w203 w230 w237 w257 w271 w280 w289 w298 w316 w328 w341 w358 w374 w401 w428 w433 w461 w483 w507 w519 w533 w547 w561 w575 w601] -> w196
          tunnel: [TRUE ("Discard?") _ _ _ _ _ _ _ _ _ _ _ _ _ _ _ _ _ _ _ _ _ _ _ _ _] -> w199
          tunnel: w198 -> [w202 w206 w229 w240 w267 w270 w279 w288 w297 w309 w330 w349 w366 w384 w390 w416 w450 w478 w504 w516 w521 w535 w549 w563 w586 w600]
          tunnel: [w202 w204 w229 w238 w265 w270 w279 w288 w297 w307 w329 w348 w364 w382 w389 w415 w444 w477 w500 w506 w520 w534 w548 w562 w585 w599] -> w195
          tunnel: w197 -> [w201 w205 w231 w255 w269 w273 w282 w291 w299 w313 w331 w351 w365 w381 w398 w417 w449 w459 w491 w518 w523 w537 w551 w565 w590 w605]
          tunnel: w193 -> [_ w209 _ _ _ _ _ _ _ _ _ _ _ _ _ _ _ _ _ _ _ _ _ _ _ _]
          event Panel Close? {
            n77 = event-data() -> ()  [unwired: 1 in, 1 out]
            n78 = event-data() -> ()  [unwired: 2 in, 1 out]
          }
          event Timeout {
            n79 = event-data() -> ()  [unwired: 1 in, 1 out]
            n80 = Unbundle By Name(w209) -> ("Vapour Generator.Type"=w208:T29, "Vapour Generator.Connection"=w207:bool)
            n81 = case shown="\"Owlstone GEN-SYS\", Default" w208 {
              tunnel: w207 -> [w214]
              tunnel: w206 -> [w213]
              tunnel: w205 -> [w212]
              tunnel: [w211] -> w204
              tunnel: [w210] -> w203
              frame "Owlstone GEN-SYS", Default {
                n82 = case shown="True" w214 {
                  tunnel: w213 -> [w216 w219]
                  tunnel: w212 -> [w215 w223]
                  tunnel: [w216 w218] -> w211
                  tunnel: [w215 w217] -> w210
                  frame False {
                  }
                  frame True {
                    n83 = Unbundle By Name(w219) -> ("Vapour Generator"=w226:refnum<class "Vapour Generator.lvclass">)
                    n84 = To More Specific Class(target class=refnum<class "Owlstone GEN-SYS.lvclass"> refnum ("Owlstone GEN-SYS.lvclass"), reference=w226) -> (specific class reference=w224:refnum<class "Owlstone GEN-SYS.lvclass">)  [unwired: 1 in, 1 out]
                    n85 = call-dynamic "Get Gas Output.vi"("error in"=w223, "Owlstone OVG-4 in"=w224) -> ("error out"=w222:errorcluster, "Output"=w221:T3, "Owlstone OVG-4 out"=w220:refnum<class "Owlstone GEN-SYS.lvclass">)  [unwired: 7 in]
                    n86 = Bundle By Name(cluster=w219, "Vapour Generator"=w220) -> (w218:T1)
                    n87 = property on="Gas Output" class="Clust (strict)"(error in=w222, "Value"=w221) -> (error out=w217:errorcluster)  [unwired: 1 in, 1 out]
                  }
                }
              }
            }
          }
          event Value Change {
            n88 = event-data() -> ()  [unwired: 1 in, 1 out]
            n89 = call "Device Params Global.vi"("action"=Device_Params_Global."Get Device Settings", "error in"=w231) -> ("error out"=w234:errorcluster, "Device Settings OUT"=w233:T31)  [unwired: 7 in, 1 out]
            n90 = Bundle By Name(cluster=w233, "PID.B-M PID"="B-M PID Settings", "PID.INL PID"="INL PID Settings") -> (w232:T31)
            n91 = call "Device Params Global.vi"("action"=Device_Params_Global."Set Device Settings", "error in"=w234, "Device Settings IN"=w232) -> ("error out"=w230:errorcluster)  [unwired: 6 in, 2 out]
          }
          event "Power Supply Apply": Value Change {
            n92 = event-data() -> ()  [unwired: 1 in, 1 out]
            n93 = Unbundle By Name(w240) -> ("Power Supply"=w256:refnum<class "Power Supply.lvclass">)
            n94 = property on="Power Supply Source Mode" class="Enum (strict)"(error in=w255) -> (error out=w254:errorcluster, "Value"=w246:T13)  [unwired: 1 in, 1 out]
            n95 = call-dynamic "Write Source Mode.vi"("error in (no error)"=w254, "Source Mode"=w246, "Power Supply in"=w256) -> ("error out"=w253:errorcluster, "Power Supply out"=w251:refnum<class "Power Supply.lvclass">)  [unwired: 7 in]
            n96 = property on="Power Supply Limits" class="Clust (strict)"(error in=w253) -> (error out=w252:errorcluster, "Value"=w250:T9)  [unwired: 1 in, 1 out]
            n97 = call-dynamic "Write Limits.vi"("error in (no error)"=w252, "Limits"=w250, "Power Supply in"=w251) -> ("error out"=w249:errorcluster, "Power Supply out"=w248:refnum<class "Power Supply.lvclass">)  [unwired: 7 in]
            n98 = call-dynamic "Set Limits.vi"("error in (no error)"=w249, "Power Supply in"=w248) -> ("error out"=w245:errorcluster, "Power Supply out"=w247:refnum<class "Power Supply.lvclass">)  [unwired: 8 in]
            n99 = property on="Power Supply Source Value" class="DigNum (strict)"(error in=w245) -> (error out=w243:errorcluster, "Value"=w244:dbl)  [unwired: 1 in, 1 out]
            n100 = property on="Power Supply Source Value Units" class="Enum (strict)"(error in=w243) -> (error out=w242:errorcluster, "Value"=w241:T12)  [unwired: 1 in, 1 out]
            n101 = call-dynamic "Set Source Value.vi"("error in (no error)"=w242, "Source Value Units"=w241, "Source Value"=w244, "Power Supply in"=w247) -> ("error out"=w237:errorcluster, "Power Supply out"=w239:refnum<class "Power Supply.lvclass">)  [unwired: 6 in]
            n102 = Bundle By Name(cluster=w240, "Power Supply"=w239) -> (w238:T1)
          }
          event "Power Supply Output": Value Change {
            n103 = event-data() -> ("NewVal"=w258:bool)  [unwired: 1 in]
            n104 = Unbundle By Name(w267) -> ("Power Supply"=w268:refnum<class "Power Supply.lvclass">)
            n105 = call-dynamic "Set Output.vi"("error in (no error)"=w269, "Enable"=w258, "Power Supply in"=w268) -> ("error out"=w259:errorcluster, "Power Supply out"=w266:refnum<class "Power Supply.lvclass">)  [unwired: 7 in]
            n106 = Bundle By Name(cluster=w267, "Power Supply"=w266) -> (w265:T1)
            n107 = call "Device Params Global.vi"("action"=Device_Params_Global."Get Device Settings", "error in"=w259) -> ("error out"=w262:errorcluster, "Device Settings OUT"=w261:T31)  [unwired: 7 in, 1 out]
            n108 = Bundle By Name(cluster=w261, "Power Supply.Output"=w258) -> (w260:T31)
            n109 = call "Device Params Global.vi"("action"=Device_Params_Global."Set Device Settings", "error in"=w262, "Device Settings IN"=w260) -> ("error out"=w257:errorcluster)  [unwired: 6 in, 2 out]
          }
          event Value Change {
            n110 = event-data() -> ("NewVal"=w272:T9)  [unwired: 1 in]
            n111 = call "Device Params Global.vi"("action"=Device_Params_Global."Get Device Settings", "error in"=w273) -> ("error out"=w276:errorcluster, "Device Settings OUT"=w275:T31)  [unwired: 7 in, 1 out]
            n112 = Bundle By Name(cluster=w275, "Power Supply.Limits"=w272) -> (w274:T31)
            n113 = call "Device Params Global.vi"("action"=Device_Params_Global."Set Device Settings", "error in"=w276, "Device Settings IN"=w274) -> ("error out"=w271:errorcluster)  [unwired: 6 in, 2 out]
          }
          event Value Change {
            n114 = event-data() -> ("NewVal"=w281:T13)  [unwired: 1 in]
            n115 = call "Device Params Global.vi"("action"=Device_Params_Global."Get Device Settings", "error in"=w282) -> ("error out"=w285:errorcluster, "Device Settings OUT"=w284:T31)  [unwired: 7 in, 1 out]
            n116 = Bundle By Name(cluster=w284, "Power Supply.Source Mode"=w281) -> (w283:T31)
            n117 = call "Device Params Global.vi"("action"=Device_Params_Global."Set Device Settings", "error in"=w285, "Device Settings IN"=w283) -> ("error out"=w280:errorcluster)  [unwired: 6 in, 2 out]
          }
          event "Power Supply Source Value": Value Change {
            n118 = event-data() -> ("NewVal"=w290:dbl)  [unwired: 1 in]
            n119 = call "Device Params Global.vi"("action"=Device_Params_Global."Get Device Settings", "error in"=w291) -> ("error out"=w294:errorcluster, "Device Settings OUT"=w293:T31)  [unwired: 7 in, 1 out]
            n120 = Bundle By Name(cluster=w293, "Power Supply.Source Value"=w290) -> (w292:T31)
            n121 = call "Device Params Global.vi"("action"=Device_Params_Global."Set Device Settings", "error in"=w294, "Device Settings IN"=w292) -> ("error out"=w289:errorcluster)  [unwired: 6 in, 2 out]
          }
          event Value Change {
            n122 = event-data() -> ("NewVal"=w300:T12)  [unwired: 1 in]
            n123 = call "Device Params Global.vi"("action"=Device_Params_Global."Get Device Settings", "error in"=w299) -> ("error out"=w303:errorcluster, "Device Settings OUT"=w302:T31)  [unwired: 7 in, 1 out]
            n124 = Bundle By Name(cluster=w302, "Power Supply.Source Value Units"=w300) -> (w301:T31)
            n125 = call "Device Params Global.vi"("action"=Device_Params_Global."Set Device Settings", "error in"=w303, "Device Settings IN"=w301) -> ("error out"=w298:errorcluster)  [unwired: 6 in, 2 out]
          }
          event Value Change {
            n126 = event-data() -> ("NewVal"=w315:T15)  [unwired: 1 in]
            n127 = Unbundle By Name(w309) -> ("Multimeter"=w314:refnum<class "Multimeter.lvclass">)
            n128 = To More Specific Class(target class=refnum<class "Agilent 3458A.lvclass"> refnum ("Agilent 3458A.lvclass"), reference=w314, error in=w313) -> (specific class reference=w311:refnum<class "Agilent 3458A.lvclass">, error out=w310:errorcluster)
            n129 = call-dynamic "Set Measurement Configuration.vi"("error in (no error)"=w310, "Measurement Configuration"=w315, "Agilent 3458A in"=w311) -> ("error out"=w306:errorcluster, "Agilent 3458A out"=w308:refnum<class "Agilent 3458A.lvclass">)  [unwired: 7 in]
            n130 = Bundle By Name(cluster=w309, "Multimeter"=w308) -> (w307:T1)
            n131 = call "Device Params Global.vi"("action"=Device_Params_Global."Get Device Settings", "error in"=w306) -> ("error out"=w319:errorcluster, "Device Settings OUT"=w318:T31)  [unwired: 7 in, 1 out]
            n132 = Bundle By Name(cluster=w318, "Multimeter.Agilent 3458A.Measurement Configuration"=w315) -> (w317:T31)
            n133 = call "Device Params Global.vi"("action"=Device_Params_Global."Set Device Settings", "error in"=w319, "Device Settings IN"=w317) -> ("error out"=w316:errorcluster)  [unwired: 6 in, 2 out]
          }
          event Value Change {
            n134 = event-data() -> ("NewVal"=w323:T14)  [unwired: 1 in]
            n135 = Unbundle By Name(w330) -> ("Multimeter"=w333:refnum<class "Multimeter.lvclass">)
            n136 = Unbundle By Name(w323) -> ("Power Line Cycles"=w322:dbl)
            n137 = To More Specific Class(target class=refnum<class "Agilent 3458A.lvclass"> refnum ("Agilent 3458A.lvclass"), reference=w333, error in=w331) -> (specific class reference=w327:refnum<class "Agilent 3458A.lvclass">, error out=w326:errorcluster)
            n138 = call-dynamic "Set Integration Time.vi"("error in (no error)"=w326, "Integration Time"=w322, "Agilent 3458A in"=w327) -> ("error out"=w325:errorcluster, "Agilent 3458A out"=w324:refnum<class "Agilent 3458A.lvclass">)  [unwired: 7 in]
            n139 = Bundle By Name(cluster=w330, "Multimeter"=w324) -> (w329:T1)
            n140 = call "Device Params Global.vi"("action"=Device_Params_Global."Get Device Settings", "error in"=w325) -> ("error out"=w336:errorcluster, "Device Settings OUT"=w335:T31)  [unwired: 7 in, 1 out]
            n141 = Bundle By Name(cluster=w335, "Multimeter.Agilent 3458A.Measurement Integration"=w323) -> (w334:T31)
            n142 = call "Device Params Global.vi"("action"=Device_Params_Global."Set Device Settings", "error in"=w336, "Device Settings IN"=w334) -> ("error out"=w328:errorcluster)  [unwired: 6 in, 2 out]
          }
          event Value Change {
            n143 = event-data() -> ("NewVal"=w342:i32)  [unwired: 1 in]
            n144 = Unbundle By Name(w349) -> ("Vapour Generator"=w354:refnum<class "Vapour Generator.lvclass">)
            n145 = To More Specific Class(target class=refnum<class "Owlstone GEN-SYS.lvclass"> refnum ("Owlstone GEN-SYS.lvclass"), reference=w354, error in=w351) -> (specific class reference=w352:refnum<class "Owlstone GEN-SYS.lvclass">, error out=w350:errorcluster)
            n146 = call "Set Oven Temperature.vi"("error in"=w350, "Oven Temperature"=w342, "OVG In"=w352) -> ("error out"=w339:errorcluster, "OVG Out"=w340:refnum<class "Owlstone GEN-SYS.lvclass">)  [unwired: 7 in]
            n147 = Bundle By Name(cluster=w349, "Vapour Generator"=w340) -> (w348:T1)
            n148 = call "Device Params Global.vi"("action"=Device_Params_Global."Get Device Settings", "error in"=w339) -> ("error out"=w345:errorcluster, "Device Settings OUT"=w344:T31)  [unwired: 7 in, 1 out]
            n149 = Bundle By Name(cluster=w344, "Vapour Generator.Owlstone GEN-SYS Setpoints.OVG-4.Oven Temperature"=w342) -> (w343:T31)
            n150 = call "Device Params Global.vi"("action"=Device_Params_Global."Set Device Settings", "error in"=w345, "Device Settings IN"=w343) -> ("error out"=w341:errorcluster)  [unwired: 6 in, 2 out]
          }
          event Value Change {
            n151 = event-data() -> ("NewVal"=w357:i32)  [unwired: 1 in]
            n152 = Unbundle By Name(w366) -> ("Vapour Generator"=w370:refnum<class "Vapour Generator.lvclass">)
            n153 = To More Specific Class(target class=refnum<class "Owlstone GEN-SYS.lvclass"> refnum ("Owlstone GEN-SYS.lvclass"), reference=w370, error in=w365) -> (specific class reference=w368:refnum<class "Owlstone GEN-SYS.lvclass">, error out=w367:errorcluster)
            n154 = call "Set Sample Flow Rate.vi"("error in"=w367, "Sample Flow"=w357, "OVG In"=w368) -> ("error out"=w355:errorcluster, "OVG Out"=w356:refnum<class "Owlstone GEN-SYS.lvclass">)  [unwired: 7 in]
            n155 = Bundle By Name(cluster=w366, "Vapour Generator"=w356) -> (w364:T1)
            n156 = call "Device Params Global.vi"("action"=Device_Params_Global."Get Device Settings", "error in"=w355) -> ("error out"=w361:errorcluster, "Device Settings OUT"=w360:T31)  [unwired: 7 in, 1 out]
            n157 = Bundle By Name(cluster=w360, "Vapour Generator.Owlstone GEN-SYS Setpoints.OVG-4.Sample Flow Rate"=w357) -> (w359:T31)
            n158 = call "Device Params Global.vi"("action"=Device_Params_Global."Set Device Settings", "error in"=w361, "Device Settings IN"=w359) -> ("error out"=w358:errorcluster)  [unwired: 6 in, 2 out]
          }
          event Value Change {
            n159 = event-data() -> ("NewVal"=w373:i32)  [unwired: 1 in]
            n160 = Unbundle By Name(w384) -> ("Vapour Generator"=w386:refnum<class "Vapour Generator.lvclass">)
            n161 = To More Specific Class(target class=refnum<class "Owlstone GEN-SYS.lvclass"> refnum ("Owlstone GEN-SYS.lvclass"), reference=w386, error in=w381) -> (specific class reference=w383:refnum<class "Owlstone GEN-SYS.lvclass">, error out=w380:errorcluster)
            n162 = call "Set Wet Air Flow Rate.vi"("error in"=w380, "Wet Air Flow Rate (ml/min)"=w373, "OVG In"=w383) -> ("error out"=w371:errorcluster, "OVG Out"=w372:refnum<class "Owlstone GEN-SYS.lvclass">)  [unwired: 7 in]
            n163 = Bundle By Name(cluster=w384, "Vapour Generator"=w372) -> (w382:T1)
            n164 = call "Device Params Global.vi"("action"=Device_Params_Global."Get Device Settings", "error in"=w371) -> ("error out"=w377:errorcluster, "Device Settings OUT"=w376:T31)  [unwired: 7 in, 1 out]
            n165 = Bundle By Name(cluster=w376, "Vapour Generator.Owlstone GEN-SYS Setpoints.OHG-4.Wet Air Flow"=w373) -> (w375:T31)
            n166 = call "Device Params Global.vi"("action"=Device_Params_Global."Set Device Settings", "error in"=w377, "Device Settings IN"=w375) -> ("error out"=w374:errorcluster)  [unwired: 6 in, 2 out]
          }
          event Value Change {
            n167 = event-data() -> ("NewVal"=w394:u16)  [unwired: 1 in]
            n168 = Unbundle By Name(w390) -> ("Vapour Generator"=w400:refnum<class "Vapour Generator.lvclass">)
            n169 = To More Specific Class(target class=refnum<class "Owlstone GEN-SYS.lvclass"> refnum ("Owlstone GEN-SYS.lvclass"), reference=w400, error in=w398) -> (specific class reference=w397:refnum<class "Owlstone GEN-SYS.lvclass">, error out=w396:errorcluster)
            n170 = call-dynamic "Read Setpoints.vi"("error in (no error)"=w396, "Owlstone GEN-SYS in"=w397) -> ("error out"=w392:errorcluster, "Setpoints"=w395:T4, "Owlstone GEN-SYS out"=w391:refnum<class "Owlstone GEN-SYS.lvclass">)  [unwired: 7 in]
            n171 = Bundle By Name(cluster=w395, "OVG-4.Split Flow Status"=w394) -> (w393:T4)
            n172 = call-dynamic "Write Setpoints.vi"("error in (no error)"=w392, "Setpoints"=w393, "Owlstone GEN-SYS in"=w391) -> ("error out"=w387:errorcluster, "Owlstone GEN-SYS out"=w388:refnum<class "Owlstone GEN-SYS.lvclass">)  [unwired: 7 in]
            n173 = Equal?(x=w394, y=u16 0) -> (x = y?=w410:bool)
            n174 = Bundle By Name(cluster=w390, "Vapour Generator"=w388) -> (w389:T1)
            n175 = Select(t=T32."Disabled and Grayed Out" ("Disabled"), s=w410, f=T32."Enabled" ("Disabled")) -> (s? t:f=w408:T32)
            n176 = property on="Split Flow Rate" class="Slide (strict)"(error in=w387, "DisabledEnum"=w408) -> (error out=w403:errorcluster)  [unwired: 1 in, 1 out]
            n177 = call "Device Params Global.vi"("action"=Device_Params_Global."Get Device Settings", "error in"=w403) -> ("error out"=w406:errorcluster, "Device Settings OUT"=w405:T31)  [unwired: 7 in, 1 out]
            n178 = Bundle By Name(cluster=w405, "Vapour Generator.Owlstone GEN-SYS Setpoints.OVG-4.Split Flow Status"=w394) -> (w404:T31)
            n179 = call "Device Params Global.vi"("action"=Device_Params_Global."Set Device Settings", "error in"=w406, "Device Settings IN"=w404) -> ("error out"=w401:errorcluster)  [unwired: 6 in, 2 out]
          }
          event Value Change {
            n180 = event-data() -> ("NewVal"=w418:i32)  [unwired: 1 in]
            n181 = Unbundle By Name(w416) -> ("Vapour Generator"=w426:refnum<class "Vapour Generator.lvclass">)
            n182 = To More Specific Class(target class=refnum<class "Owlstone GEN-SYS.lvclass"> refnum ("Owlstone GEN-SYS.lvclass"), reference=w426, error in=w417) -> (specific class reference=w424:refnum<class "Owlstone GEN-SYS.lvclass">, error out=w423:errorcluster)
            n183 = call-dynamic "Read Setpoints.vi"("error in (no error)"=w423, "Owlstone GEN-SYS in"=w424) -> ("error out"=w420:errorcluster, "Setpoints"=w422:T4, "Owlstone GEN-SYS out"=w419:refnum<class "Owlstone GEN-SYS.lvclass">)  [unwired: 7 in]
            n184 = Bundle By Name(cluster=w422, "OVG-4.Split Flow Rate"=w418) -> (w421:T4)
            n185 = call-dynamic "Write Setpoints.vi"("error in (no error)"=w420, "Setpoints"=w421, "Owlstone GEN-SYS in"=w419) -> ("error out"=w413:errorcluster, "Owlstone GEN-SYS out"=w414:refnum<class "Owlstone GEN-SYS.lvclass">)  [unwired: 7 in]
            n186 = Bundle By Name(cluster=w416, "Vapour Generator"=w414) -> (w415:T1)
            n187 = call "Device Params Global.vi"("action"=Device_Params_Global."Get Device Settings", "error in"=w413) -> ("error out"=w431:errorcluster, "Device Settings OUT"=w430:T31)  [unwired: 7 in, 1 out]
            n188 = Bundle By Name(cluster=w430, "Vapour Generator.Owlstone GEN-SYS Setpoints.OVG-4.Split Flow Rate"=w418) -> (w429:T31)
            n189 = call "Device Params Global.vi"("action"=Device_Params_Global."Set Device Settings", "error in"=w431, "Device Settings IN"=w429) -> ("error out"=w428:errorcluster)  [unwired: 6 in, 2 out]
          }
          event Value Change {
            n190 = event-data() -> ("NewVal"=w455:T6)  [unwired: 1 in]
            n191 = Unbundle By Name(w450) -> ("Vapour Generator"=w448:refnum<class "Vapour Generator.lvclass">)
            n192 = To More Specific Class(target class=refnum<class "Owlstone GEN-SYS.lvclass"> refnum ("Owlstone GEN-SYS.lvclass"), reference=w448) -> (specific class reference=w447:refnum<class "Owlstone GEN-SYS.lvclass">)  [unwired: 1 in, 1 out]
            n193 = call-dynamic "Set Tube Parameters.vi"("error in (no error)"=w449, "Tube Gas"=w455, "Owlstone GEN-SYS in"=w447) -> ("error out"=w434:errorcluster, "Calibration Temperature"=w437:i32, "Permeation Rate"=w454:i32, "Owlstone GEN-SYS out"=w435:refnum<class "Owlstone GEN-SYS.lvclass">, "Molecular Weight"=w451:dbl)  [unwired: 4 in]
            n194 = Bundle By Name(cluster=w450, "Vapour Generator"=w435) -> (w444:T1)
            n195 = property on="Permeation Rate \n(ng/min)" class="DigNum (strict)"(error in=w434, "Value"=w454) -> (error out=w453:errorcluster)  [unwired: 1 in, 1 out]
            n196 = property on="Calibration Temperature\n(Celcius)" class="DigNum (strict)"(error in=w453, "Value"=w437) -> (error out=w452:errorcluster)  [unwired: 1 in, 1 out]
            n197 = property on="Molecular Weight" class="DigNum (strict)"(error in=w452, "Value"=w451) -> (error out=w445:errorcluster)  [unwired: 1 in, 1 out]
            n198 = property on="Owlstone Permeation Tube" class="Clust (strict)"(error in=w445) -> (error out=w436:errorcluster, "Value"=w440:T39)  [unwired: 1 in, 1 out]
            n199 = call "Device Params Global.vi"("action"=Device_Params_Global."Get Device Settings", "error in"=w436) -> ("error out"=w438:errorcluster, "Device Settings OUT"=w441:T31)  [unwired: 7 in, 1 out]
            n200 = Bundle By Name(cluster=w441, "Vapour Generator.Owlstone Permeation Tube"=w440) -> (w439:T31)
            n201 = call "Device Params Global.vi"("action"=Device_Params_Global."Set Device Settings", "error in"=w438, "Device Settings IN"=w439) -> ("error out"=w433:errorcluster)  [unwired: 6 in, 2 out]
          }
          event Value Change {
            n202 = event-data() -> ("NewVal"=w460:T16)  [unwired: 1 in]
            n203 = Unbundle By Name(w478) -> ("Mass Flow Controller"=w468:refnum<class "Mass Flow Controller.lvclass">)
            n204 = property on="MFC Flow Rate" class="Slide (strict)"(error in=w459) -> (error out=w457:errorcluster, "Value"=w474:T17)  [unwired: 1 in, 1 out]
            n205 = call-dynamic "Set Valve Status.vi"("Valve Status"=w460, "error in (no error)"=w459, "Mass Flow Controller in"=w468) -> ("error out"=w458:errorcluster, "Mass Flow Controller out"=w479:refnum<class "Mass Flow Controller.lvclass">)  [unwired: 7 in]
            n206 = To Variant(anything=w474) -> (Variant=w473:variant)
            n207 = To Variant(anything=w460) -> (Variant=w472:variant)
            n208 = Bundle By Name(cluster=w478, "Mass Flow Controller"=w479) -> (w477:T1)
            n209 = Build Array(w473, w472) -> (w470:variant[])
            n210 = Merge Errors(w458, w457) -> (w456:errorcluster)
            n211 = call "Status Bar.vi"("action"=Status_Bar."Insert Into Status Bar", "error in"=w456, "Parameters"=w470, "Devices"=Devices."Mass Flow Controller") -> ("error out"=w471:errorcluster)  [unwired: 6 in, 1 out]
            n212 = call "User Interface Global.vi"("error in"=w471, "action"=User_Interface_Action."Status Bar Set") -> ("error out"=w462:errorcluster)  [unwired: 9 in]
            n213 = call "Device Params Global.vi"("action"=Device_Params_Global."Get Device Settings", "error in"=w462) -> ("error out"=w465:errorcluster, "Device Settings OUT"=w464:T31)  [unwired: 7 in, 1 out]
            n214 = Bundle By Name(cluster=w464, "Mass Flow Controller.MFC Valve Status"=w460) -> (w463:T31)
            n215 = call "Device Params Global.vi"("action"=Device_Params_Global."Set Device Settings", "error in"=w465, "Device Settings IN"=w463) -> ("error out"=w461:errorcluster)  [unwired: 6 in, 2 out]
          }
          event Value Change {
            n216 = event-data() -> ("NewVal"=w484:T17)  [unwired: 1 in]
            n217 = Unbundle By Name(w504) -> ("Mass Flow Controller"=w503:refnum<class "Mass Flow Controller.lvclass">)
            n218 = call-dynamic "Set Flow Rate.vi"("error in (no error)"=w491, "Flow Rate Units"=Flow_Rate_Units."ml/min", "Flow Rate"=w484, "Mass Flow Controller in"=w503) -> ("error out"=w482:errorcluster, "Mass Flow Controller out"=w502:refnum<class "Mass Flow Controller.lvclass">)  [unwired: 6 in]
            n219 = property on="MFC Valve Status" class="Enum (strict)"(error in=w491) -> (error out=w480:errorcluster, "Value"=w493:T16)  [unwired: 1 in, 1 out]
            n220 = Bundle By Name(cluster=w504, "Mass Flow Controller"=w502) -> (w500:T1)
            n221 = Merge Errors(w482, w480) -> (w481:errorcluster)
            n222 = To Variant(anything=w484) -> (Variant=w495:variant)
            n223 = To Variant(anything=w493) -> (Variant=w494:variant)
            n224 = Build Array(w495, w494) -> (w492:variant[])
            n225 = call "Status Bar.vi"("action"=Status_Bar."Insert Into Status Bar", "error in"=w481, "Parameters"=w492, "Devices"=Devices."Mass Flow Controller") -> ("error out"=w497:errorcluster)  [unwired: 6 in, 1 out]
            n226 = call "User Interface Global.vi"("error in"=w497, "action"=User_Interface_Action."Status Bar Set") -> ("error out"=w485:errorcluster)  [unwired: 9 in]
            n227 = call "Device Params Global.vi"("action"=Device_Params_Global."Get Device Settings", "error in"=w485) -> ("error out"=w488:errorcluster, "Device Settings OUT"=w487:T31)  [unwired: 7 in, 1 out]
            n228 = Bundle By Name(cluster=w487, "Mass Flow Controller.MFC Flow Rate"=w484) -> (w486:T31)
            n229 = call "Device Params Global.vi"("action"=Device_Params_Global."Set Device Settings", "error in"=w488, "Device Settings IN"=w486) -> ("error out"=w483:errorcluster)  [unwired: 6 in, 2 out]
          }
          event Value Change {
            w505 = T40 1 items=["Valve 1"=1, "Valve 2"=2, "Valve 3"=3, "Valve 4"=4, "Valve 5"=5, "Valve 6"=6, "Valve 7"=7] ("valve in")
            n230 = event-data() -> ("NewVal"=w509:T19)  [unwired: 1 in]
            n231 = Unbundle By Name(w516) -> ("Valve Controller"=w517:refnum<class "Valve Controller.lvclass">)
            n232 = call-dynamic "Set.vi"("error in (no error)"=w518, "status in"=w509, "valve in"=w505, "Valve Controller in"=w517) -> ("error out"=w508:errorcluster, "Valve Controller out"=w515:refnum<class "Valve Controller.lvclass">)  [unwired: 4 in, 2 out]
            n233 = Bundle By Name(cluster=w516, "Valve Controller"=w515) -> (w506:T1)
            n234 = call "Device Params Global.vi"("action"=Device_Params_Global."Get Device Settings", "error in"=w508) -> ("error out"=w512:errorcluster, "Device Settings OUT"=w511:T31)  [unwired: 7 in, 1 out]
            n235 = Bundle By Name(cluster=w511, "Valve Controller.Valve Assembly.Valve 1"=w509) -> (w510:T31)
            n236 = call "Device Params Global.vi"("action"=Device_Params_Global."Set Device Settings", "error in"=w512, "Device Settings IN"=w510) -> ("error out"=w507:errorcluster)  [unwired: 6 in, 2 out]
          }
          event Value Change {
            w524 = T40 2 items=["Valve 1"=1, "Valve 2"=2, "Valve 3"=3, "Valve 4"=4, "Valve 5"=5, "Valve 6"=6, "Valve 7"=7] ("valve in")
            n237 = event-data() -> ("NewVal"=w522:T19)  [unwired: 1 in]
            n238 = Unbundle By Name(w521) -> ("Valve Controller"=w532:refnum<class "Valve Controller.lvclass">)
            n239 = call-dynamic "Set.vi"("error in (no error)"=w523, "status in"=w522, "valve in"=w524, "Valve Controller in"=w532) -> ("error out"=w525:errorcluster, "Valve Controller out"=w531:refnum<class "Valve Controller.lvclass">)  [unwired: 4 in, 2 out]
            n240 = Bundle By Name(cluster=w521, "Valve Controller"=w531) -> (w520:T1)
            n241 = call "Device Params Global.vi"("action"=Device_Params_Global."Get Device Settings", "error in"=w525) -> ("error out"=w528:errorcluster, "Device Settings OUT"=w527:T31)  [unwired: 7 in, 1 out]
            n242 = Bundle By Name(cluster=w527, "Valve Controller.Valve Assembly.Valve 2"=w522) -> (w526:T31)
            n243 = call "Device Params Global.vi"("action"=Device_Params_Global."Set Device Settings", "error in"=w528, "Device Settings IN"=w526) -> ("error out"=w519:errorcluster)  [unwired: 6 in, 2 out]
          }
          event Value Change {
            w538 = T40 3 items=["Valve 1"=1, "Valve 2"=2, "Valve 3"=3, "Valve 4"=4, "Valve 5"=5, "Valve 6"=6, "Valve 7"=7] ("valve in")
            n244 = event-data() -> ("NewVal"=w536:T19)  [unwired: 1 in]
            n245 = Unbundle By Name(w535) -> ("Valve Controller"=w546:refnum<class "Valve Controller.lvclass">)
            n246 = call-dynamic "Set.vi"("error in (no error)"=w537, "status in"=w536, "valve in"=w538, "Valve Controller in"=w546) -> ("error out"=w539:errorcluster, "Valve Controller out"=w545:refnum<class "Valve Controller.lvclass">)  [unwired: 4 in, 2 out]
            n247 = Bundle By Name(cluster=w535, "Valve Controller"=w545) -> (w534:T1)
            n248 = call "Device Params Global.vi"("action"=Device_Params_Global."Get Device Settings", "error in"=w539) -> ("error out"=w542:errorcluster, "Device Settings OUT"=w541:T31)  [unwired: 7 in, 1 out]
            n249 = Bundle By Name(cluster=w541, "Valve Controller.Valve Assembly.Valve 3"=w536) -> (w540:T31)
            n250 = call "Device Params Global.vi"("action"=Device_Params_Global."Set Device Settings", "error in"=w542, "Device Settings IN"=w540) -> ("error out"=w533:errorcluster)  [unwired: 6 in, 2 out]
          }
          event Value Change {
            w552 = T40 4 items=["Valve 1"=1, "Valve 2"=2, "Valve 3"=3, "Valve 4"=4, "Valve 5"=5, "Valve 6"=6, "Valve 7"=7] ("valve in")
            n251 = event-data() -> ("NewVal"=w550:T19)  [unwired: 1 in]
            n252 = Unbundle By Name(w549) -> ("Valve Controller"=w560:refnum<class "Valve Controller.lvclass">)
            n253 = call-dynamic "Set.vi"("error in (no error)"=w551, "status in"=w550, "valve in"=w552, "Valve Controller in"=w560) -> ("error out"=w553:errorcluster, "Valve Controller out"=w559:refnum<class "Valve Controller.lvclass">)  [unwired: 4 in, 2 out]
            n254 = Bundle By Name(cluster=w549, "Valve Controller"=w559) -> (w548:T1)
            n255 = call "Device Params Global.vi"("action"=Device_Params_Global."Get Device Settings", "error in"=w553) -> ("error out"=w556:errorcluster, "Device Settings OUT"=w555:T31)  [unwired: 7 in, 1 out]
            n256 = Bundle By Name(cluster=w555, "Valve Controller.Valve Assembly.Valve 4"=w550) -> (w554:T31)
            n257 = call "Device Params Global.vi"("action"=Device_Params_Global."Set Device Settings", "error in"=w556, "Device Settings IN"=w554) -> ("error out"=w547:errorcluster)  [unwired: 6 in, 2 out]
          }
          event Value Change {
            w566 = T40 5 items=["Valve 1"=1, "Valve 2"=2, "Valve 3"=3, "Valve 4"=4, "Valve 5"=5, "Valve 6"=6, "Valve 7"=7] ("valve in")
            n258 = event-data() -> ("NewVal"=w564:T19)  [unwired: 1 in]
            n259 = Unbundle By Name(w563) -> ("Valve Controller"=w574:refnum<class "Valve Controller.lvclass">)
            n260 = call-dynamic "Set.vi"("error in (no error)"=w565, "status in"=w564, "valve in"=w566, "Valve Controller in"=w574) -> ("error out"=w567:errorcluster, "Valve Controller out"=w573:refnum<class "Valve Controller.lvclass">)  [unwired: 4 in, 2 out]
            n261 = Bundle By Name(cluster=w563, "Valve Controller"=w573) -> (w562:T1)
            n262 = call "Device Params Global.vi"("action"=Device_Params_Global."Get Device Settings", "error in"=w567) -> ("error out"=w570:errorcluster, "Device Settings OUT"=w569:T31)  [unwired: 7 in, 1 out]
            n263 = Bundle By Name(cluster=w569, "Valve Controller.Valve Assembly.Valve 5"=w564) -> (w568:T31)
            n264 = call "Device Params Global.vi"("action"=Device_Params_Global."Set Device Settings", "error in"=w570, "Device Settings IN"=w568) -> ("error out"=w561:errorcluster)  [unwired: 6 in, 2 out]
          }
          event "Valves Close All": Value Change {
            w589 = T19 0 items=["Closed", "Open"] ("status in")
            w588 = T40[] [1, 2, 3, 4, 5] items=["Valve 1"=1, "Valve 2"=2, "Valve 3"=3, "Valve 4"=4, "Valve 5"=5, "Valve 6"=6, "Valve 7"=7]
            n265 = event-data() -> ()  [unwired: 1 in, 1 out]
            n266 = Unbundle By Name(w586) -> ("Valve Controller"=w591:refnum<class "Valve Controller.lvclass">)
            n267 = for {
              shift-right: [w596] -> w584
              shift-left: w590 -> [w597]
              shift-right: [w595] -> w587
              shift-left: w591 -> [w598]
              tunnel: w589 -> [w594]
              tunnel: w588 -> [w593] mode=indexing
              tunnel: [w592] -> w583 mode=indexing
              n268 = call-dynamic "Set.vi"("error in (no error)"=w597, "status in"=w594, "valve in"=w593, "Valve Controller in"=w598) -> ("error out"=w596:errorcluster, "status out"=w592:T19, "Valve Controller out"=w595:refnum<class "Valve Controller.lvclass">)  [unwired: 4 in, 1 out]
            }
            n269 = Index Array(array=w583) -> (element #1=w581:T19, element #2=w580:T19, element #3=w579:T19, element #4=w578:T19, element #5=w577:T19)  [unwired: 5 in]
            n270 = Bundle(cluster=T33 {"Valve 1"=0, "Valve 2"=0, "Valve 3"=0, "Valve 4"=0, "Valve 5"=0} ("Valve Assembly"), "Valve 1"=w581, "Valve 2"=w580, "Valve 3"=w579, "Valve 4"=w578, "Valve 5"=w577) -> (w576:T33)
            n271 = Bundle By Name(cluster=w586, "Valve Controller"=w587) -> (w585:T1)
            n272 = property on="Valve Assembly" class="Clust (strict)"(error in=w584, "Value"=w576) -> (error out=w575:errorcluster)  [unwired: 1 in, 1 out]
          }
          event "Valves Open All": Value Change {
            w614 = T19 1 items=["Closed", "Open"] ("status in")
            w613 = T40[] [1, 2, 3, 4, 5] items=["Valve 1"=1, "Valve 2"=2, "Valve 3"=3, "Valve 4"=4, "Valve 5"=5, "Valve 6"=6, "Valve 7"=7]
            n273 = event-data() -> ()  [unwired: 1 in, 1 out]
            n274 = Unbundle By Name(w600) -> ("Valve Controller"=w615:refnum<class "Valve Controller.lvclass">)
            n275 = for {
              shift-right: [w620] -> w604
              shift-left: w605 -> [w621]
              shift-right: [w619] -> w612
              shift-left: w615 -> [w622]
              tunnel: w614 -> [w618]
              tunnel: w613 -> [w617] mode=indexing
              tunnel: [w616] -> w611 mode=indexing
              n276 = call-dynamic "Set.vi"("error in (no error)"=w621, "status in"=w618, "valve in"=w617, "Valve Controller in"=w622) -> ("error out"=w620:errorcluster, "status out"=w616:T19, "Valve Controller out"=w619:refnum<class "Valve Controller.lvclass">)  [unwired: 4 in, 1 out]
            }
            n277 = Index Array(array=w611) -> (element #1=w610:T19, element #2=w609:T19, element #3=w608:T19, element #4=w607:T19, element #5=w606:T19)  [unwired: 5 in]
            n278 = Bundle(cluster=T33 {"Valve 1"=0, "Valve 2"=0, "Valve 3"=0, "Valve 4"=0, "Valve 5"=0} ("Valve Assembly"), "Valve 1"=w610, "Valve 2"=w609, "Valve 3"=w608, "Valve 4"=w607, "Valve 5"=w606) -> (w602:T33)
            n279 = Bundle By Name(cluster=w600, "Valve Controller"=w612) -> (w599:T1)
            n280 = property on="Valve Assembly" class="Clust (strict)"(error in=w604, "Value"=w602) -> (error out=w601:errorcluster)  [unwired: 1 in, 1 out]
          }
        }
      }
    }
  }
  "error out" <- w8
  "Class Objects Out" <- w6
